vi "mix_tap_light_stimuli.vi"() -> ()   [LabVIEW 2014]
panel:
  in  "Proportion with only tap":dbl
  in  "Proportion with only light":dbl
  in  "Hold light before tap (frames)":dbl
  in  "LED ON per cycle (frames)":dbl
  in  "Period per cycle(frames)":dbl
  in  "Light power (uW/mm^2)":i32
  in  "Taps per cycle (count)":i32
  in  "Total duration (frames)":dbl
  out "Frames":i32
  in  "Transfer and Run Date Folder After Experiment":bool
  in  "SSH user name":string
  in  "SSH password":string
  in  "Wait before recording (s)":dbl
  in  "Tags":string
  in  "Start Recording":bool
  # "Period for one cycle (blank +sti)"
  # "Randomly shuffle cycles into standard stimuli (LED+tap), only LED and only tap"
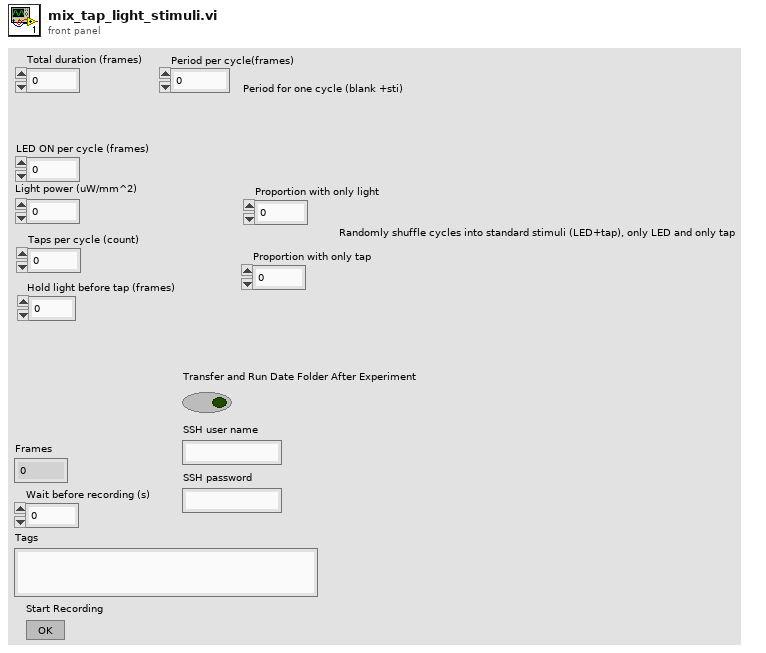
[diagram p1: front panel]
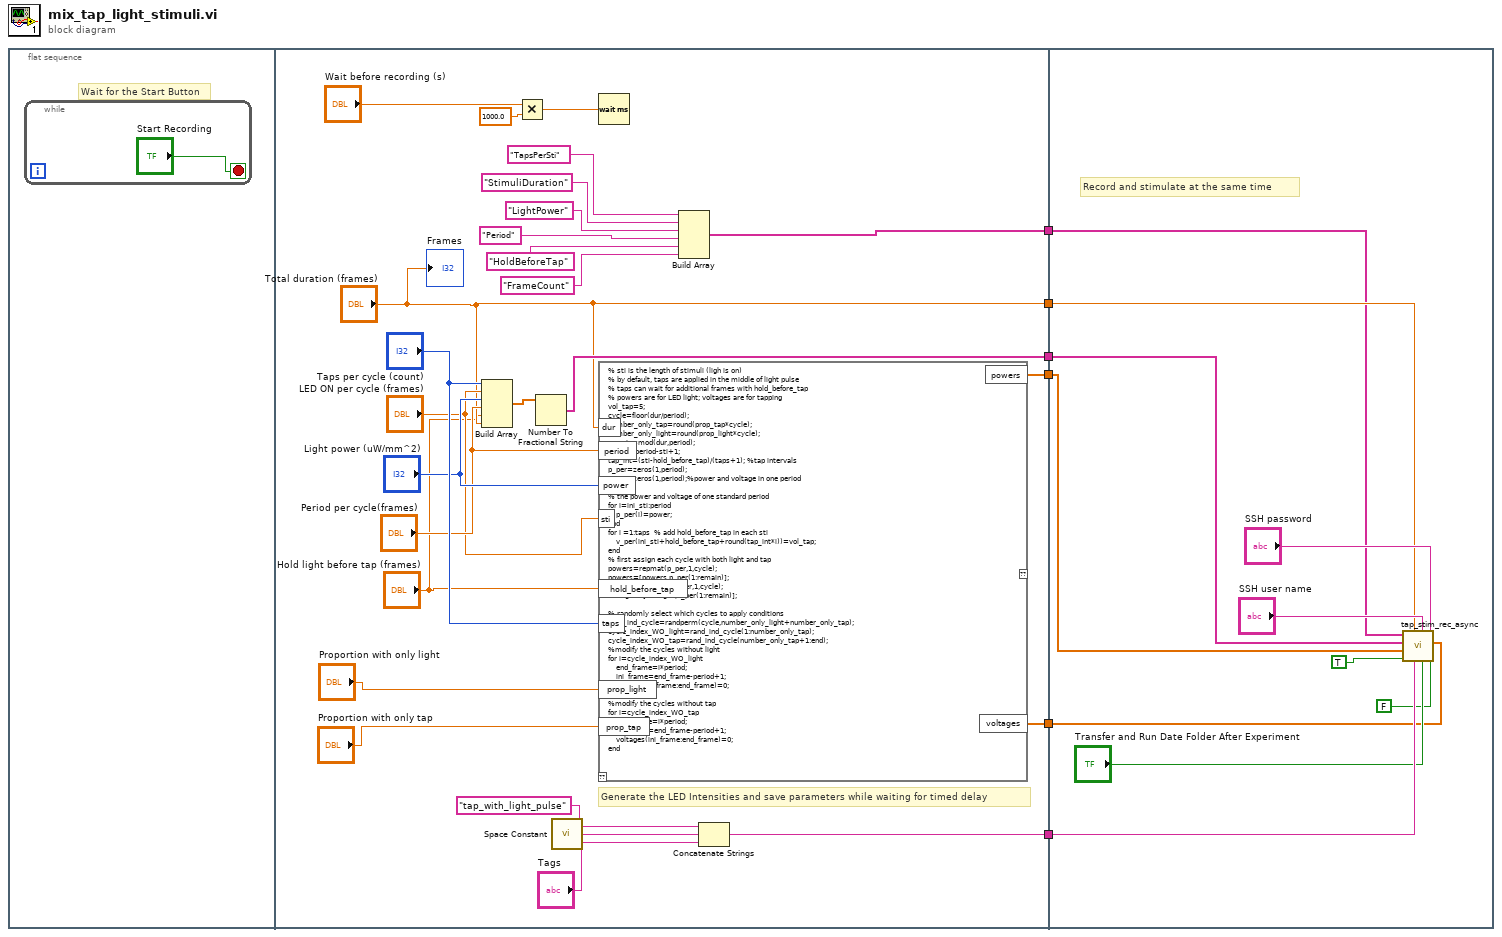
[diagram p0: block diagram]
diagram:
  n1 = flat-sequence {
    tunnel: [w30] -> w6
    tunnel: [w21] -> w5
    tunnel: ["Total duration (frames)"] -> w4
    tunnel: [w19] -> w3
    tunnel: [w15] -> w2
    tunnel: [w14] -> w1
    tunnel: w6 -> [w44]
    tunnel: w5 -> [w36]
    tunnel: w4 -> [w40]
    tunnel: w3 -> [w39]
    tunnel: w2 -> [w35]
    tunnel: w1 -> [w34]
    frame #0 {
      # "Wait for the Start Button"
      n2 = while {
        stop <- "Start Recording" stop-if-true
      }
    }
    frame #1 {
      # "Generate the LED Intensities and save parameters while waiting for timed delay"
      n3 = Build Array("Taps per cycle (count)", "LED ON per cycle (frames)", "Light power (uW/mm^2)", "Period per cycle(frames)", "Hold light before tap (frames)", "Total duration (frames)") -> (w20:dbl[])
      n4 = Multiply(x="Wait before recording (s)", y=1000.0) -> (x*y=w28:dbl)
      n5 = Number To Fractional String(number=w20) -> (F-format string=w14:string[])  [unwired: 3 in]
      n6 = call <vilib>:"Space Constant.vi"() -> ("String"=w32:string)
      n7 = Wait (ms)(milliseconds to wait=w28) -> ()  [unwired: 1 out]
      n8 = script code="% sti is the length of stimuli (ligh is on)\n% by default, taps are applied in the middle of light pulse\n% taps can wait for additional frames with hold_before_tap\n% powers are for LED light; voltages are for tapping\nvol_tap=5; \ncycle=floor(dur/period);\nnumber_only_tap=round(prop_tap*cycle);\nnumber_only_light=round(prop_light*cycle);\nremain=mod(dur,period);\nini_sti=period-sti+1;\ntap_int=(sti-hold_before_tap)/(taps+1); %tap intervals\np_per=zeros(1,period);\nv_per=zeros(1,period);%power and voltage in one period\n\n% the power and voltage of one standard period\nfor i=ini_sti:period  \n    p_per(i)=power;\nend\nfor i =1:taps  % add hold_before_tap in each sti\n    v_per(ini_sti+hold_before_tap+round(tap_int*i))=vol_tap; \nend\n% first assign each cycle with both light and tap\npowers=repmat(p_per,1,cycle);\npowers=[powers,p_per(1:remain)]; \nvoltages =repmat(v_per,1,cycle);\nvoltages=[voltages,v_per(1:remain)];\n\n% randomly select which cycles to apply conditions \nrand_ind_cycle=randperm(cycle,number_only_light+number_only_tap);\ncycle_index_WO_light=rand_ind_cycle(1:number_only_tap);\ncycle_index_WO_tap=rand_ind_cycle(number_only_tap+1:end);\n%modify the cycles without light\nfor i=cycle_index_WO_light\n    end_frame=i*period;\n    ini_frame=end_frame-period+1;\n    powers(ini_frame:end_frame)=0;\nend\n%modify the cycles without tap\nfor i=cycle_index_WO_tap\n    end_frame=i*period;\n    ini_frame=end_frame-period+1;\n    voltages(ini_frame:end_frame)=0;\nend"("power"="Light power (uW/mm^2)", "taps"="Taps per cycle (count)", "sti"="LED ON per cycle (frames)", "period"="Period per cycle(frames)", "dur"="Total duration (frames)", "hold_before_tap"="Hold light before tap (frames)", "prop_light"="Proportion with only light", "prop_tap"="Proportion with only tap") -> ("powers"=w19:dbl[], "voltages"=w15:dbl[])  [unwired: 1 in, 1 out]
      n9 = Build Array("TapsPerSti", "StimuliDuration", "LightPower", "Period", "HoldBeforeTap", "FrameCount") -> (w21:string[])
      n10 = Concatenate Strings("tap_with_light_pulse", w32, "Tags") -> (w30:string)
      "Frames" <- "Total duration (frames)"
    }
    frame #2 {
      # "Record and stimulate at the same time"
      n11 = call "tap_stim_rec_async.vi"("Convert Power to Voltage B"=FALSE, "voltages/power B"=w35, "SSH password"="SSH password", "Transfer and Run Date Folder After Experiment"="Transfer and Run Date Folder After Experiment", "SSH user name"="SSH user name", "Tags"=w44, "Frames"=w40, "Convert Power to Voltage A"=TRUE, "voltages/power A"=w39, "parameters"=w34, "parameters headers"=w36) -> ()  [unwired: 1 in]
    }
  }
